vi "Receiver.vi"() -> ()   [LabVIEW 2013]
uses:
  <instrlib>/niUSRP/niUSRP Fetch Rx Data (CDB Cluster).vi
  <vilib>/addons/Modulation/niDMT.lvlib
panel:
  in  "Packet Parameters":T1={"Message Bits"=128, "Sync Bits"=20, "Guard Bits "=30, "Number of Packets to Expect"=46}
  out "Correct Packets Rx":i16=25000
  in  "Matching Filter Parameters":T2={"Alpha"=0.5, "Filter Length"=6, "TX Filter"=enum."Root Raised Cos"} {"Alpha" format="%.2f"}
  out "Signal & Noise Power":cluster{"noise_power":dbl, "signal_power":dbl}={"noise_power"=2.571229598792933e-12, "signal_power"=1.4546950663593878e-09}
  out "Actual Rx Parameters":T3={"Rx IQ Sampling\nRate [s/sec]"=400000.0, "Rx Frequency [Hz]"=915000000.0, "Rx Gain [dB]"=20.0, "Rx Antenna"=""} {"Rx Gain [dB]" format="%#.6p"; "Rx Frequency [Hz]" format="%#.6p"; "Rx IQ Sampling\nRate [s/sec]" format="%#.6p"}
  in  "Rx Parameters":T3={"Rx IQ Sampling\nRate [s/sec]"=400000.0, "Rx Frequency [Hz]"=915000000.0, "Rx Gain [dB]"=20.0, "Rx Antenna"=""} {"Rx Gain [dB]" format="%#.6p"; "Rx Frequency [Hz]" format="%#.6p"; "Rx IQ Sampling\nRate [s/sec]" format="%#.6p"}
  in  "USRP IP Address":refnum<k15>="192.168.10.2"
  in  "Modulation Type":string(combo)="QPSK"
  out "Constellation Graph":T4(graph)
  out "Received Signal":dbl[](graph)
  out "Error Out":errorcluster={"status"=FALSE, "code"=1074118647, "source"="niUSRP Fetch Rx Data (CDB Cluster).vi<ERR>Overflow: an internal receive buffer has filled before the data could be returned.  Consider reducing the IQ rate, increasing the Fetch rate, or increasing the number of samples per Fetch."}
  out "Symbol Rate [symbols/sec]":dbl=25000.0 format="%#.6p"
  in  "PN Sequence Order for Sync":i32=31
  in  "Stop":bool
  out "Sync Found":bool
  out "Recovered Message":string
  in  "Acquisition Duration [sec]":dbl=0.04 format="%#.6p"
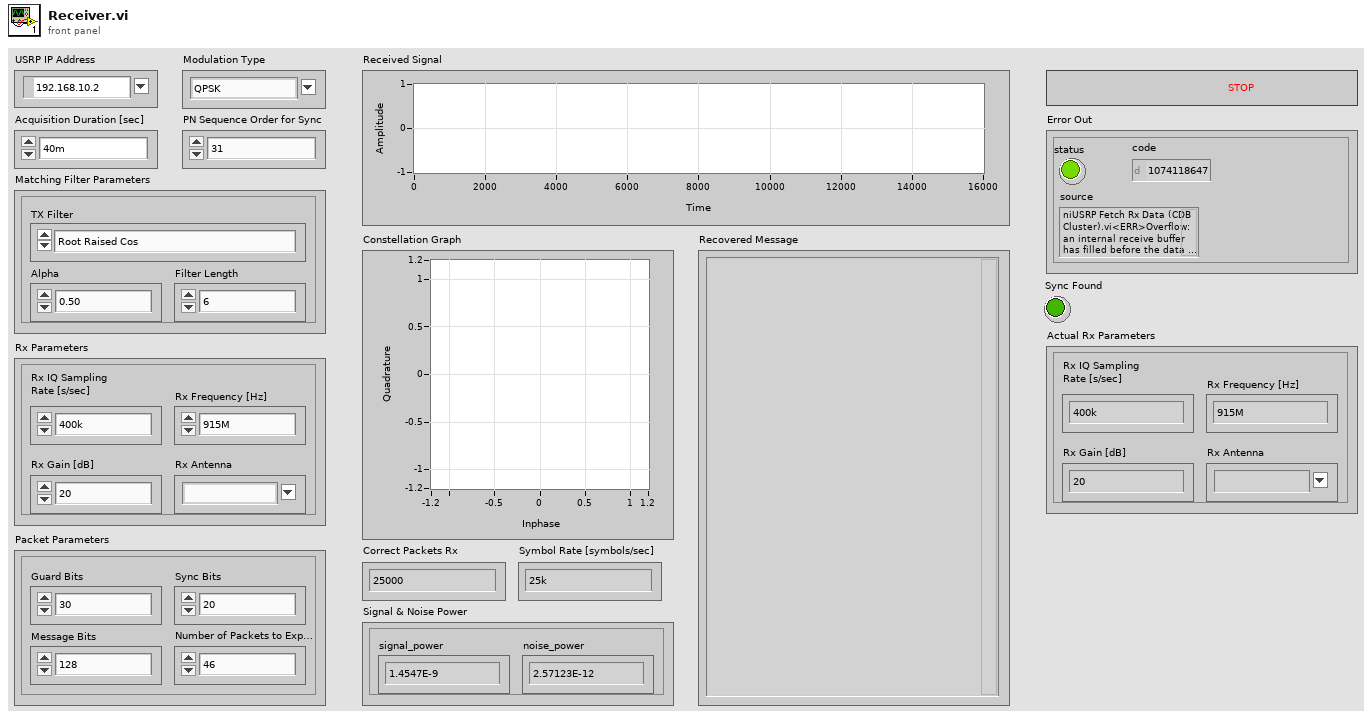
[diagram p1: front panel]
types:
  T1 = cluster{"Message Bits":i32, "Sync Bits":i32, "Guard Bits ":i32, "Number of Packets to Expect":i32}
  T2 = cluster{"Alpha":dbl, "Filter Length":i32, "TX Filter":enum16{"none", "Raised Cosine", "Root Raised Cos", "Gaussian"}}
  T3 = cluster{"Rx IQ Sampling\nRate [s/sec]":dbl, "Rx Frequency [Hz]":dbl, "Rx Gain [dB]":dbl, "Rx Antenna":string}
  T4 = cluster{"constellation":dbl[], "oversampled data":dbl[]}[]
  T5 = cluster{"expected sync location (symbols)":i32, "sync sequence":cdb[], "sync location uncertainty (symbols)":i32, "sync indent (symbols)":i32}
  T6 = cluster{"Packet Array":i32[][], "IP Array of Pkt Nums Received  ":bool[]}
  T7 = cluster{"bit stream ":i8[][], "Sync Valid?":bool[], "Decoded Pkt Numbers":u32[], "Enable?":bool}
  T8 = cluster{"packet_arr":cdb[][], "Packets Valid?":bool}
  T9 = cluster{"PSK type":u16, "Samples per Symbol":i32, "Differential PSK":enum16{"disable", "enable"}, "M":i32}
  T10 = cluster{"Rx IQ Sampling\nRate [s/sec]":dbl, "Rx\nFrequency [Hz]":dbl, "Rx Gain [dB]":dbl, "Rx Antenna":string}
  T11 = cluster{"PSK system parameters":cluster{"samples per symbol (16)":i32, "symbol map":cdb[], "differential PSK":enum16{"disable", "enable"}, "PSK type":u16}, "pulse shaping filter coefficients":dbl[], "matched filter coefficients":dbl[], "synchronization parameters":cluster{"expected sync location (symbols)":i32, "sync sequence":cdb[], "sync location uncertainty (symbols)":i32, "sync indent (symbols)":i32}, "Sync Bits":i8[]}
  T12 = typedef "niAMT.lvlib/Complex Data Waveform.ctl" = cluster{"t0":dbl, "dt":dbl, "Y":cdb[]}
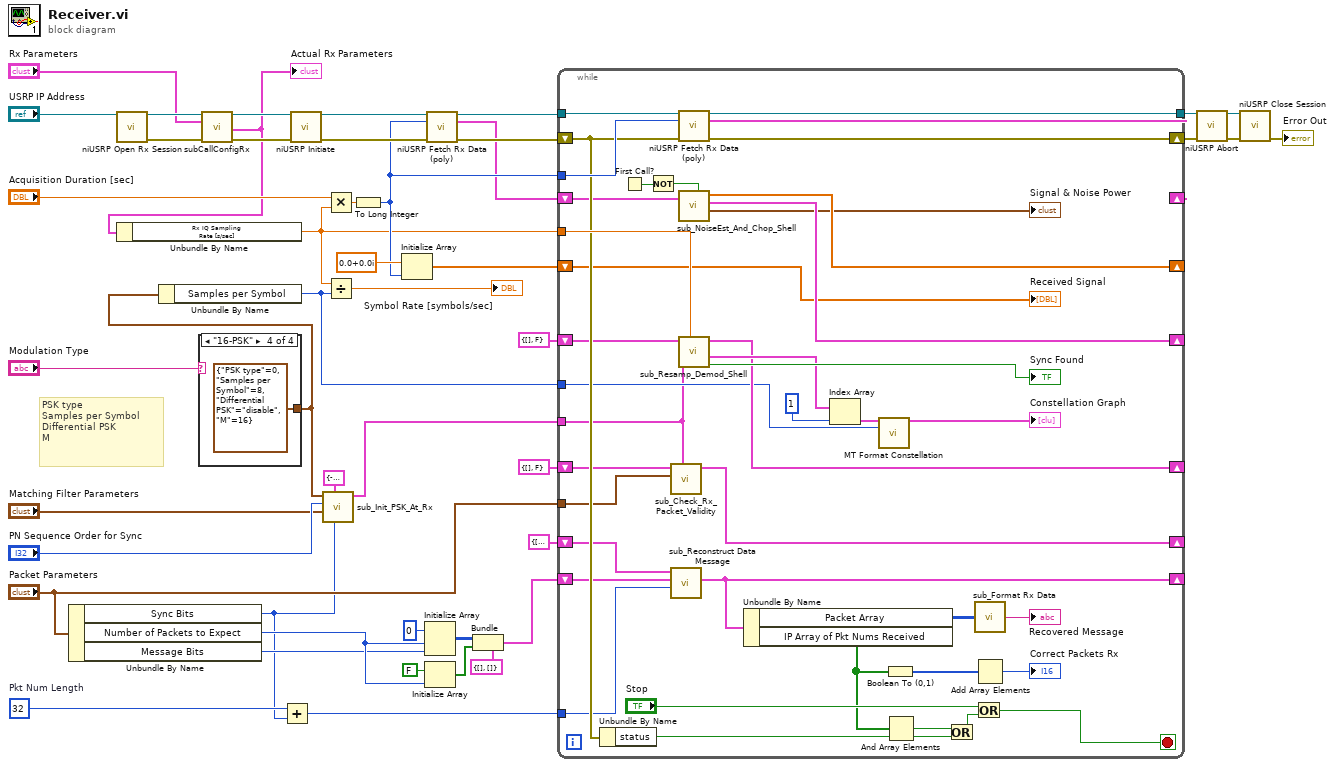
[diagram p0: block diagram]
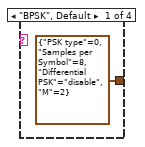
[diagram p2: hidden frame]
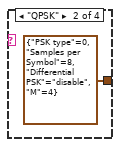
[diagram p3: hidden frame]
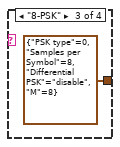
[diagram p4: hidden frame]
diagram:
  w31 = 32  # Pkt Num Length
  # "PSK type\nSamples per Symbol\nDifferential PSK\nM"
  n1 = Unbundle By Name("Packet Parameters") -> ("Sync Bits"=w4:i32, "Number of Packets to Expect"=w6:i32, "Message Bits"=w5:i32)
  n2 = call <instrlib>:"niUSRP Open Rx Session.vi"("device names"="USRP IP Address") -> ("session handle out"=w43:refnum<k15>, "error out"=w44:errorcluster)  [unwired: 13 in]
  n3 = case shown="\"16-PSK\"" "Modulation Type" {
    tunnel: [T9 {"PSK type"=0, "Samples per Symbol"=8, "Differential PSK"=enum."disable", "M"=2} ("PSK Parameters") T9 {"PSK type"=0, "Samples per Symbol"=8, "Differential PSK"=enum."disable", "M"=4} ("PSK Parameters") T9 {"PSK type"=0, "Samples per Symbol"=8, "Differential PSK"=enum."disable", "M"=8} ("PSK Parameters") T9 {"PSK type"=0, "Samples per Symbol"=8, "Differential PSK"=enum."disable", "M"=16} ("PSK Parameters")] -> w1
    frame "BPSK", Default {
    }
    frame "QPSK" {
    }
    frame "8-PSK" {
    }
    frame "16-PSK" {
    }
  }
  n4 = Unbundle By Name(w1) -> ("Samples per Symbol"=w8:i32)
  n5 = call "subCallConfigRx.vi"("session handle"=w43, "Rx Parameters"="Rx Parameters", "error in"=w44) -> ("session handle out"=w42:refnum<k15>, "Actual Rx Parameters"=w10:T10, "error out"=w41:errorcluster)  [unwired: 10 in]
  "Actual Rx Parameters" <- w10
  n6 = Unbundle By Name(w10) -> ("Rx IQ Sampling\nRate [s/sec]"=w13:dbl)
  n7 = Add(x=w31, y=w4) -> (x+y=w34:i32)
  n8 = call <instrlib>:"niUSRP Initiate.vi"("session handle"=w42, "error in (no error)"=w41) -> ("session handle out"=w19:refnum<k15>, "error out"=w18:errorcluster)  [unwired: 12 in]
  n9 = call "sub_Init_PSK_At_Rx.vi"("Sync Bits"=w4, "synchronization parameters"=T5 {"expected sync location (symbols)"=-1, "sync sequence"=[], "sync location uncertainty (symbols)"=0, "sync indent (symbols)"=0}, "filter parameters"="Matching Filter Parameters", "PN sequence order (9)"="PN Sequence Order for Sync", "PSK Parameters"=w1) -> ("PSK Init Parameters"=w33:T11)  [unwired: 5 in, 1 out]
  n10 = Multiply(x="Acquisition Duration [sec]", y=w13) -> (x*y=w46:dbl)
  n11 = Divide(x=w13, y=w8) -> (x/y=→"Symbol Rate [symbols/sec]":dbl)
  n12 = To Long Integer(number=w46) -> (32bit integer=w17:i32)
  n13 = Initialize Array(cdb 0.0+0.0i ("element"), w17) -> (w24:cdb[])
  n14 = Initialize Array(0, w6, w5) -> (w26:i32[][])
  n15 = Initialize Array(FALSE, w6) -> (w25:bool[])
  n16 = call-poly <instrlib>:"niUSRP Fetch Rx Data (poly).vi"("session handle"=w19, "number of samples"=w17, "error in (no error)"=w18) -> ("session handle out"=w21:refnum<k15>, "data"=w16:cluster{"t0":dbl, "dt":dbl, "Y":cdb[]}, "error out"=w20:errorcluster)  [unwired: 9 in, 1 out]
  n17 = Bundle(cluster=T6 {"Packet Array"=[], "IP Array of Pkt Nums Received  "=[]} ("Packet Info"), "Packet Array"=w26, "IP Array of Pkt Nums Received"=w25) -> (w14:T6)
  n18 = while {
    tunnel: w13 -> [w90]
    tunnel: w21 -> [w80]
    tunnel: [w78] -> w38
    tunnel: w17 -> [w77]
    tunnel: "Packet Parameters" -> [w51]
    tunnel: w34 -> [w64]
    tunnel: w33 -> [w58]
    shift-right: [w79] -> w37
    shift-left: w20 -> [w75]
    tunnel: w8 -> [w59]
    shift-right: [w62] -> _
    shift-left: w14 -> [w65]
    shift-right: [w71] -> _
    shift-left: T8 {"packet_arr"=[], "Packets Valid?"=FALSE} -> [w72]
    shift-right: [w67] -> _
    shift-left: cluster{"bit stream":i8[][], "Enable?":bool} {"bit stream"=[], "Enable?"=FALSE} ("Output Bitstream") -> [w70]
    shift-right: [w57] -> _
    shift-left: T7 {"bit stream "=[], "Sync Valid?"=[], "Decoded Pkt Numbers"=[], "Enable?"=FALSE} ("Output Bit Stream") -> [w66]
    shift-right: [w68] -> _
    shift-left: w16 -> [w69]
    shift-right: [w60] -> _
    shift-left: w24 -> [w56]
    stop <- w52 stop-if-true
    n19 = Unbundle By Name(w75) -> ("status"=w74:bool)
    n20 = First Call?() -> (First Call?: T/F=w82:bool)
    n21 = Not(x=w82) -> (.not. x?=w81:bool)
    n22 = call "sub_Check_Rx_Packet_Validity.vi"("PSK Init Parameters"=w58, "Packet Parameters"=w51, "Input Bit Stream"=w70) -> ("Output Bit Stream"=w57:T7)  [unwired: 7 in]
    n23 = call "sub_Reconstruct Data Message.vi"("Start Loc of Data"=w64, "Packet Info"=w65, "Input Stream"=w66) -> ("Packet Info out"=w62:T6)  [unwired: 8 in]
    n24 = call-poly <instrlib>:"niUSRP Fetch Rx Data (poly).vi"("session handle"=w80, "number of samples"=w77, "error in (no error)"=w75) -> ("session handle out"=w78:refnum<k15>, "data"=w68:cluster{"t0":dbl, "dt":dbl, "Y":cdb[]}, "error out"=w79:errorcluster)  [unwired: 9 in, 1 out]
    n25 = call "sub_NoiseEst_And_Chop_Shell.vi"("data"=w69, "Enable"=w81) -> ("Singal & Noise Power"=→"Signal & Noise Power":cluster{"signal_power":dbl, "noise_power":dbl}, "Output Packets"=w71:cluster{"Packets":cdb[][], "Enable?":bool}, "Delay signal (for plotting use only)"=w60:cdb[])  [unwired: 3 in]
    n26 = call "sub_Resamp_Demod_Shell.vi"("Rx IQ Sampling\nRate [s/sec]"=w90, "PSK Init Parameters"=w58, "Input Packets"=w72) -> ("Synch Found?"=→"Sync Found":bool, "recovered complex waveform"=w85:T12[], "Output Bitstream"=w67:cluster{"bit stream":i8[][], "Enable?":bool})  [unwired: 3 in]
    n27 = Unbundle By Name(w62) -> ("Packet Array"=w63:i32[][], "IP Array of Pkt Nums Received"=w61:bool[])
    n28 = Index Array(array=w85, index=1) -> (element=w84:T12)
    n29 = call <vilib>:"MT Format Constellation.vi"("waveform"=w84, "samples per symbol"=w59) -> ("constellation graph"=→"Constellation Graph":T4)  [unwired: 3 in, 10 out]
    n30 = Boolean To (0,1)(Boolean=w61) -> (0, 1=w89:i16[])
    n31 = And Array Elements(Boolean array=w61) -> (logical AND=w76:bool)
    n32 = Or(x=w76, y=w74) -> (x .or. y?=w73:bool)
    n33 = Or(x="Stop", y=w73) -> (x .or. y?=w52:bool)
    n34 = call "sub_Format Rx Data.vi"("Output Packet Array"=w63) -> ("Received Message"=→"Recovered Message":string)
    n35 = Add Array Elements(numeric array=w89) -> (sum=→"Correct Packets Rx":i16)
    "Received Signal" <- w56
  }
  n36 = call <instrlib>:"niUSRP Abort.vi"("session handle"=w38, "error in (no error)"=w37) -> ("session handle out"=w39:refnum<k15>, "error out"=w40:errorcluster)  [unwired: 12 in]
  n37 = call <instrlib>:"niUSRP Close Session.vi"("session handle"=w39, "error in (no error)"=w40) -> ("error out"=→"Error Out":errorcluster)  [unwired: 13 in]
